vi "serverSideChatting.vi"() -> ()   [LabVIEW 2019]
panel:
  in  "Stop from Server Side":bool
  out "Data Written":i32
  out "error out":errorcluster
  in  "Message":string
  in  "Full Name":string
  in  "IsSingle":bool
  in  "Age":dbl
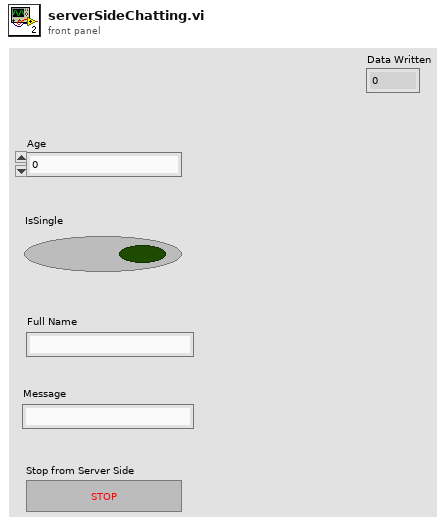
[diagram p1: front panel]
types:
  T1 = cluster{"Age ":dbl, "IsSingle":bool, "Full Name ":string, "Message ":string}
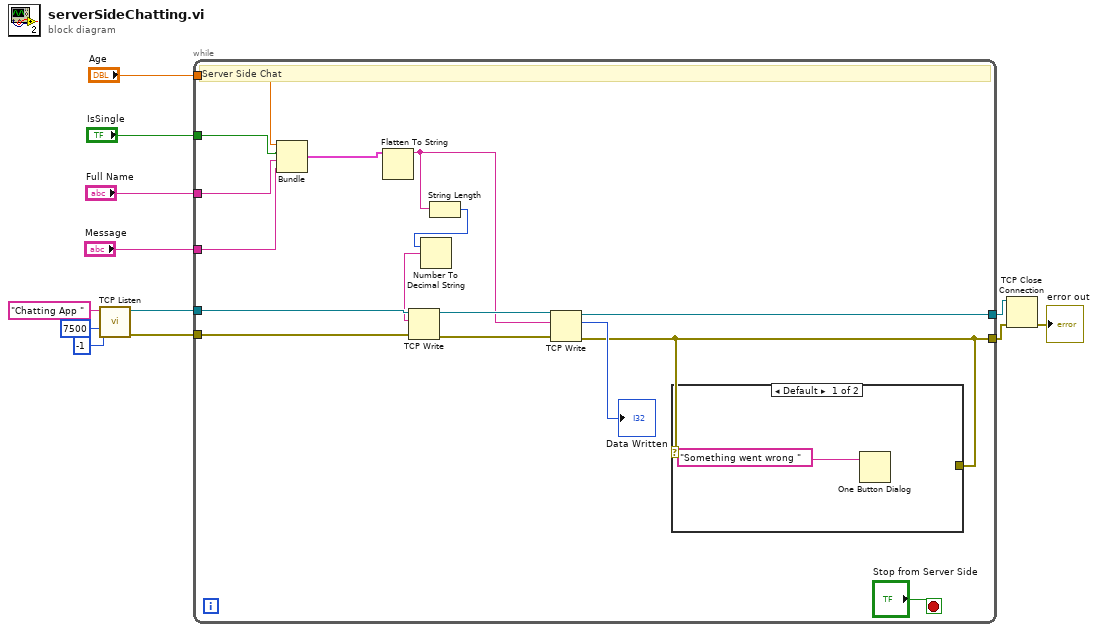
[diagram p0: block diagram]
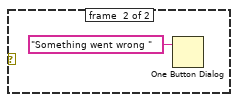
[diagram p2: hidden frame]
diagram:
  n1 = call <vilib>:"TCP Listen.vi"("timeout ms (wait forever: -1)"=-1, "port"=u16 7500, "service name"="Chatting App ") -> ("error out"=w7:errorcluster, "connection ID"=w8:refnum<k5>)  [unwired: 4 in, 3 out]
  n2 = while {
    tunnel: w8 -> [w28]
    tunnel: w7 -> [w27]
    tunnel: [w24] -> w6
    tunnel: [w13] -> w5
    tunnel: "Age" -> [w23]
    tunnel: "IsSingle" -> [w22]
    tunnel: "Full Name" -> [w21]
    tunnel: "Message" -> [w20]
    stop <- "Stop from Server Side" stop-if-true
    # "Server Side Chat"
    n3 = Bundle("Age"=w23, "IsSingle"=w22, "Full Name"=w21, "Message"=w20) -> (w19:T1)  [unwired: 1 in]
    n4 = Flatten To String(anything=w19) -> (data string=w16:string)  [unwired: 3 in, 2 out]
    n5 = String Length(string=w16) -> (length=w18:i32)
    n6 = Number To Decimal String(number=w18) -> (decimal integer string=w17:string)  [unwired: 1 in]
    n7 = TCP Write(connection ID=w28, data in=w17, error in (no error)=w27) -> (connection ID out=w25:refnum<k5>, error out=w26:errorcluster)  [unwired: 1 in, 1 out]
    n8 = TCP Write(connection ID=w25, data in=w16, error in (no error)=w26) -> (connection ID out=w24:refnum<k5>, bytes written=→"Data Written":i32, error out=w13:errorcluster)  [unwired: 1 in]
    n9 = case shown="Default" w13 {
      tunnel: w13 -> [_ _]
      frame #0 {
        n10 = One Button Dialog(message="Something went wrong ") -> ()  [unwired: 1 in, 1 out]
      }
      frame #1 {
        n11 = One Button Dialog(message="Something went wrong ") -> ()  [unwired: 1 in, 1 out]
      }
    }
  }
  n12 = TCP Close Connection(connection ID=w6, error in (no error)=w5) -> (error out=→"error out":errorcluster)  [unwired: 1 in, 1 out]
